vi "Insert Trial Timestamp to Db.vi"(8 "error in (no error)":errorcluster, 10 "Timetsamp Time":timestamp, 11 "TrialBasedExperiment in":refnum<class "TrialBasedExperiment.lvclass">) -> (0 "error out":errorcluster, 3 "TrialBasedExperiment out":refnum<class "TrialBasedExperiment.lvclass">)   [LabVIEW 2014, in "AcquisitionCoreObjects.lvlib" / "TrialBasedExperiment.lvclass"]
uses:
  TrialBasedExperiment.lvclass
  Acquisition/AcquistionObject/AcquistionObject.lvclass
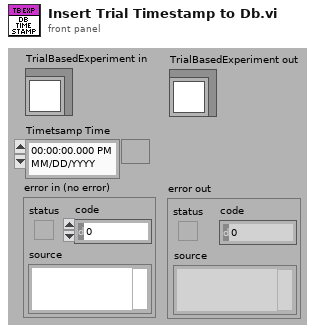
[diagram p1: front panel]
types:
  T1 = cluster{"setup":u8, "subject_id":i32, "session_start_time":dbl, "stim_start_time":dbl, "time":dbl}
  T2 = typedef "NI_Database_API.lvlib/Conn ObjectReference.ctl" = refnum<k1>
  T3 = typedef "StimulationPrimary.ctl" = cluster{"setup":u8, "subject_id":i32, "session_start_time":dbl, "stim_start_time":dbl}
  T4 = cluster{"reference":T2, "table":string, "columns":string[], i32}
  T5 = cluster{cluster{"reference":T2, "table":string, "columns":string[], i32}, "Variant":variant}
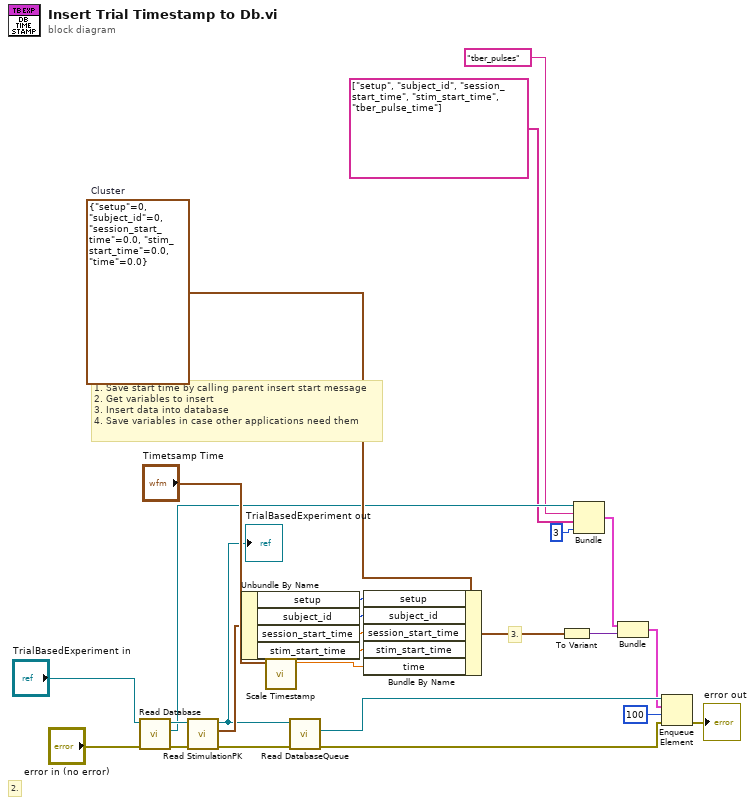
[diagram p0: block diagram]
diagram:
  w26 = T1 {"setup"=0, "subject_id"=0, "session_start_time"=0.0, "stim_start_time"=0.0, "time"=0.0}  # Cluster
  # "2."
  # "3."
  # "1. Save start time by calling parent insert start message\n2. Get variables to insert\n3. Insert data into database\n4. Save variables in case other applications need them"
  n1 = call-dynamic "Read Database.vi"("error in (no error)"="error in (no error)", "AcquistionObject in"="TrialBasedExperiment in") -> ("error out"=w18:errorcluster, "reference"=w14:T2, "AcquistionObject out"=w16:refnum<class "TrialBasedExperiment.lvclass">)  [unwired: 7 in]
  n2 = call-dynamic "Read StimulationPK.vi"("error in (no error)"=w18, "TrialBasedExperiment in"=w16) -> ("error out"=w6:errorcluster, "StimulationPK"=w17:T3, "TrialBasedExperiment out"=w11:refnum<class "TrialBasedExperiment.lvclass">)  [unwired: 7 in]
  "TrialBasedExperiment out" <- w11
  n3 = Unbundle By Name(w17) -> ("setup"=w25:u8, "subject_id"=w24:i32, "session_start_time"=w19:dbl, "stim_start_time"=w23:dbl)
  n4 = call "Scale Timestamp.vi"("Time Stamp"="Timetsamp Time") -> ("Scaled timestamp"=w21:dbl)  [unwired: 10 in]
  n5 = call-dynamic "Read DatabaseQueue.vi"("error in (no error)"=w6, "AcquistionObject in"=w11) -> ("error out"=w8:errorcluster, "DatabaseQueue"=w10:refnum<queue>)  [unwired: 7 in, 1 out]
  n6 = Bundle By Name(cluster=w26, "setup"=w25, "subject_id"=w24, "session_start_time"=w19, "stim_start_time"=w23, "time"=w21) -> (w2:T1)
  n7 = To Variant(anything=w2) -> (Variant=w3:variant)
  n8 = Bundle("reference"=w14, "table"="tber_pulses", "columns"=string[] ["setup", "subject_id", "session_start_time", "stim_start_time", "tber_pulse_time"], 3) -> (w4:T4)  [unwired: 1 in]
  n9 = Bundle(w4, "Variant"=w3) -> (w1:T5)  [unwired: 1 in]
  n10 = Enqueue Element(queue=w10, element=w1, timeout in ms (-1)=100, error in (no error)=w8) -> (error out=→"error out":errorcluster)  [unwired: 2 out]
